vi "GreaseTestingByAleks.vi"() -> ()   [LabVIEW 2021]
uses:
  <vilib>/Utility/error.llb/DialogType.ctl
  <vilib>/DAQmx/read.llb/DAQmx Read (Analog 2D DBL NChan NSamp).vi
  <vilib>/Analysis/baseanly.llb/A x Vector.vi
  <vilib>/DAQmx/create/channels.llb/DAQmx Create Channel (AI-Voltage-Basic).vi
  <vilib>/DAQmx/configure/timing.llb/DAQmx Timing (Sample Clock).vi
  <vilib>/DAQmx/miscellaneous.llb/DAQmx Fill In Error Info.vi
  <vilib>/Utility/file.llb/Write To Spreadsheet File (DBL).vi
  <vilib>/Utility/file.llb/Read Delimited Spreadsheet (string).vi
  Zaber A Series/Zaber A Series.lvlib
  <vilib>/Analysis/NI_AALBase.lvlib
panel:
  out "Force Units 2":string
  out "Torque Units 2":string
  in  "Transform":T1
  out "Calibration Matrix":dbl[][](array[numeric])
  out "Voltages":dbl[][](array[numeric])
  out "F/T":dbl[][](array[numeric]) format="%0.2f"
  out "Bias Voltages":dbl[][](array[numeric])
  out "Bias Vector":dbl[](array[numeric])
  in  "Setting":string(combo)
  out "Command Responses":string[](array[string])
  in  "Data":string
  in  "Command List":string(combo)
  in  "Value to Send":string
  out "Current Value":string
  in  "Send Command":bool
  in  "Get Setting":bool
  in  "Change Setting":bool
  in  "Torque Units":string
  in  "Force Units":string
  in  "Calibration File":path
  in  "First Channel":i16
  in  "DAQ Card":tag
  in  "Samples to Read":i32=1000
  in  "stop":bool
  out "Measurement":dbl[][](graph) caption="F/T Data"
  in  "Bias":bool
  in  "Unbias":bool
  in  "Collect Data":bool=TRUE
  in  "Data File":path
  in  "Maximum Value":dbl=10.0 format="%0.2f"
  in  "Minimum Value":dbl=-10.0 format="%0.2f"
  in  "Sample Rate":dbl=10000.0 caption="Sample Rate (Hz)" format="%0.2f"
  in  "Units (0: microsteps)":u16(ring) items=["microsteps", "microns", "millimeters", "inches"]
  in  "Device Number & Axis":string(combo)
  in  "Microstep Size (0)":dbl
  out "Device Number\n& Axis":string[](array[string])
  out "Model Name":string[](array[string])
  out "Microstep\nSize":dbl[](array[numeric])
  out "Motion Type":string[](array[string])
  in  "Move Distance (0)":dbl format="%#_12f"
  in  "Movement Type (0: relative)":u16(ring) items=["relative", "absolute"]
  in  "VISA resource name":refnum<visa-resource-name>
  in  "Start Tracking":bool
  out "Position":dbl format="%#_15f"
  in  "Identify Devices":bool
  in  "Close Port":bool
  in  "Execute Movement":bool
  in  "Home":bool
  in  "Open Port":bool
  # "Greases Control Panel"
  # "Things Aleks is Not Sure About"
  # "Force Sensor Things That Aleks Doesn't Understand"
  # "Send Command"
  # "Read and Modify Settings"
  # "Setup"
  # "Running"
  # "Motor Control Port Settings"
  # "Force Sensor DAQ Settings"
  # "Force Sensor File Settings"
  # "Force Sensor Output and Controls"
  # "Identify Connected Devices"
  # "Send Movement"
  # "Don't Collect Data"
  # "Motor Shared Settings"
  # "Force Sensor Measurement Settings"
  # "Home Devices"
  # "Position Tracking"
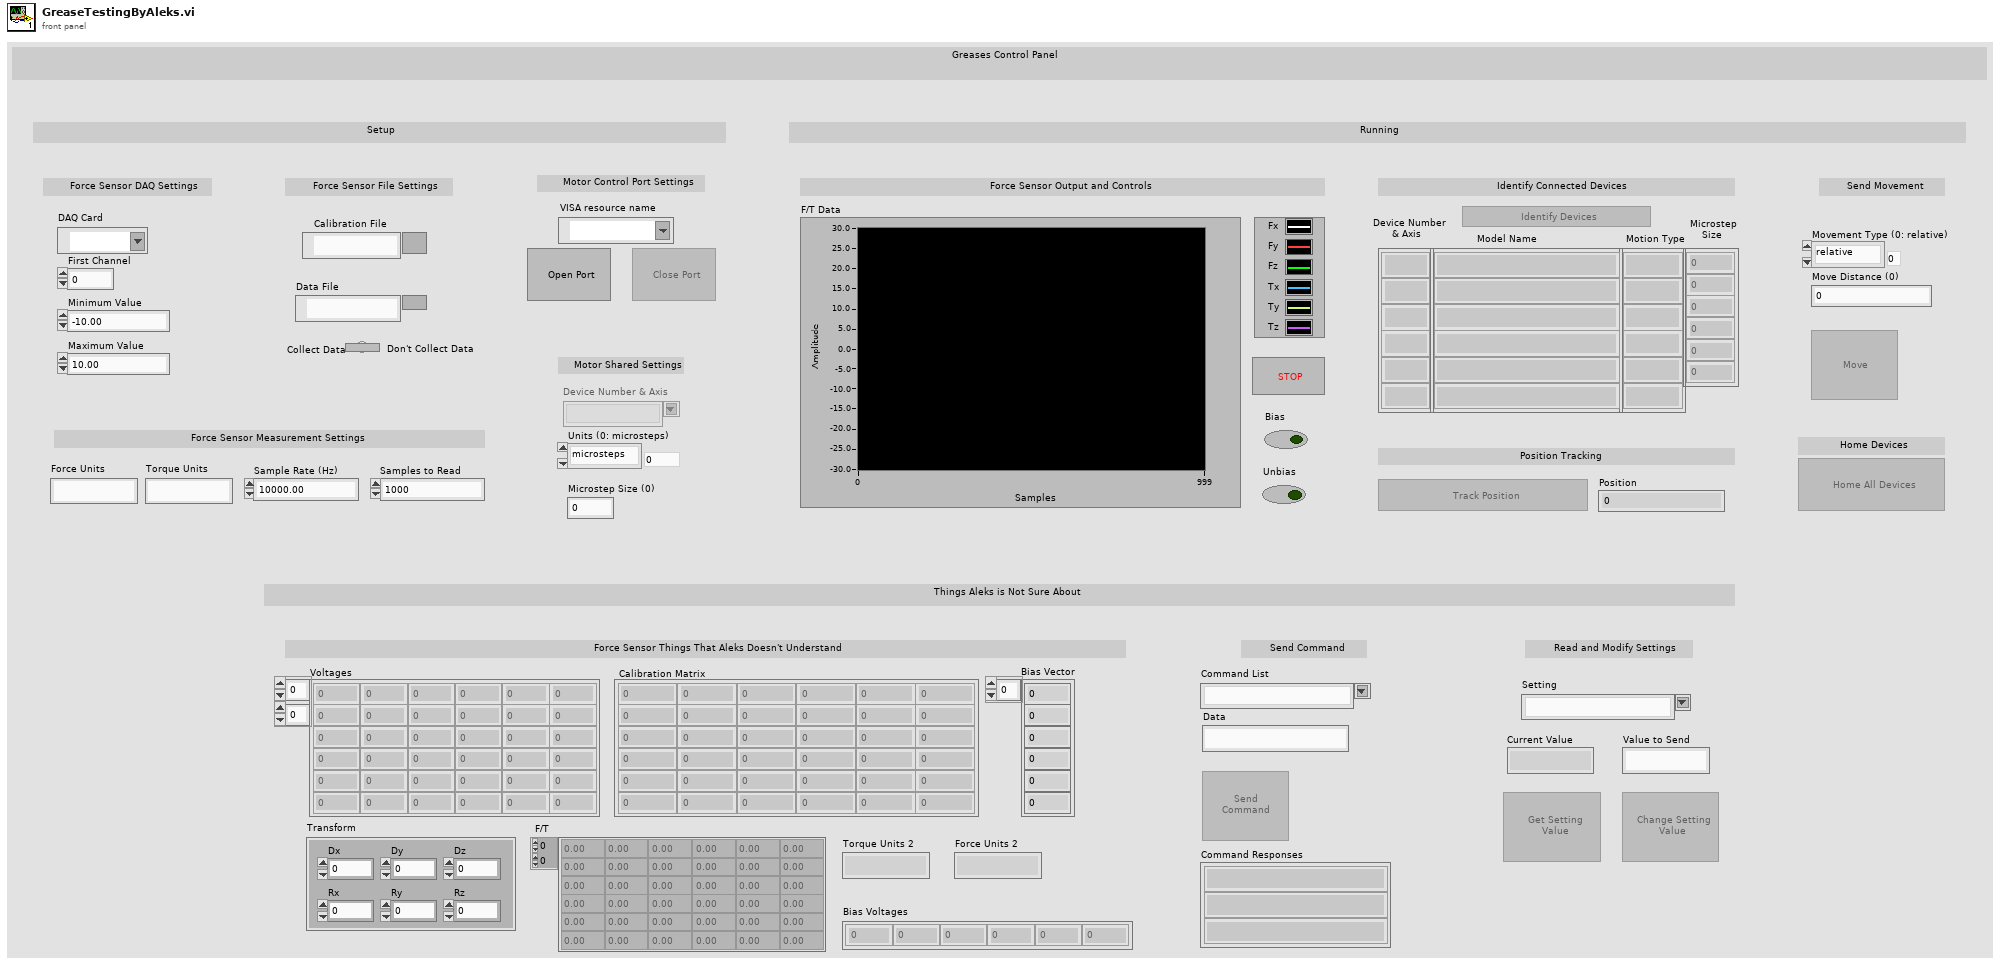
[diagram p1: front panel]
types:
  T1 = cluster{"Dx":dbl, "Dy":dbl, "Dz":dbl, "Rx":dbl, "Ry":dbl, "Rz":dbl}
  T2 = typedef "DialogType.ctl" = u16
  T3 = enum8{"Enabled", "Disabled", "Disabled and Grayed Out"}
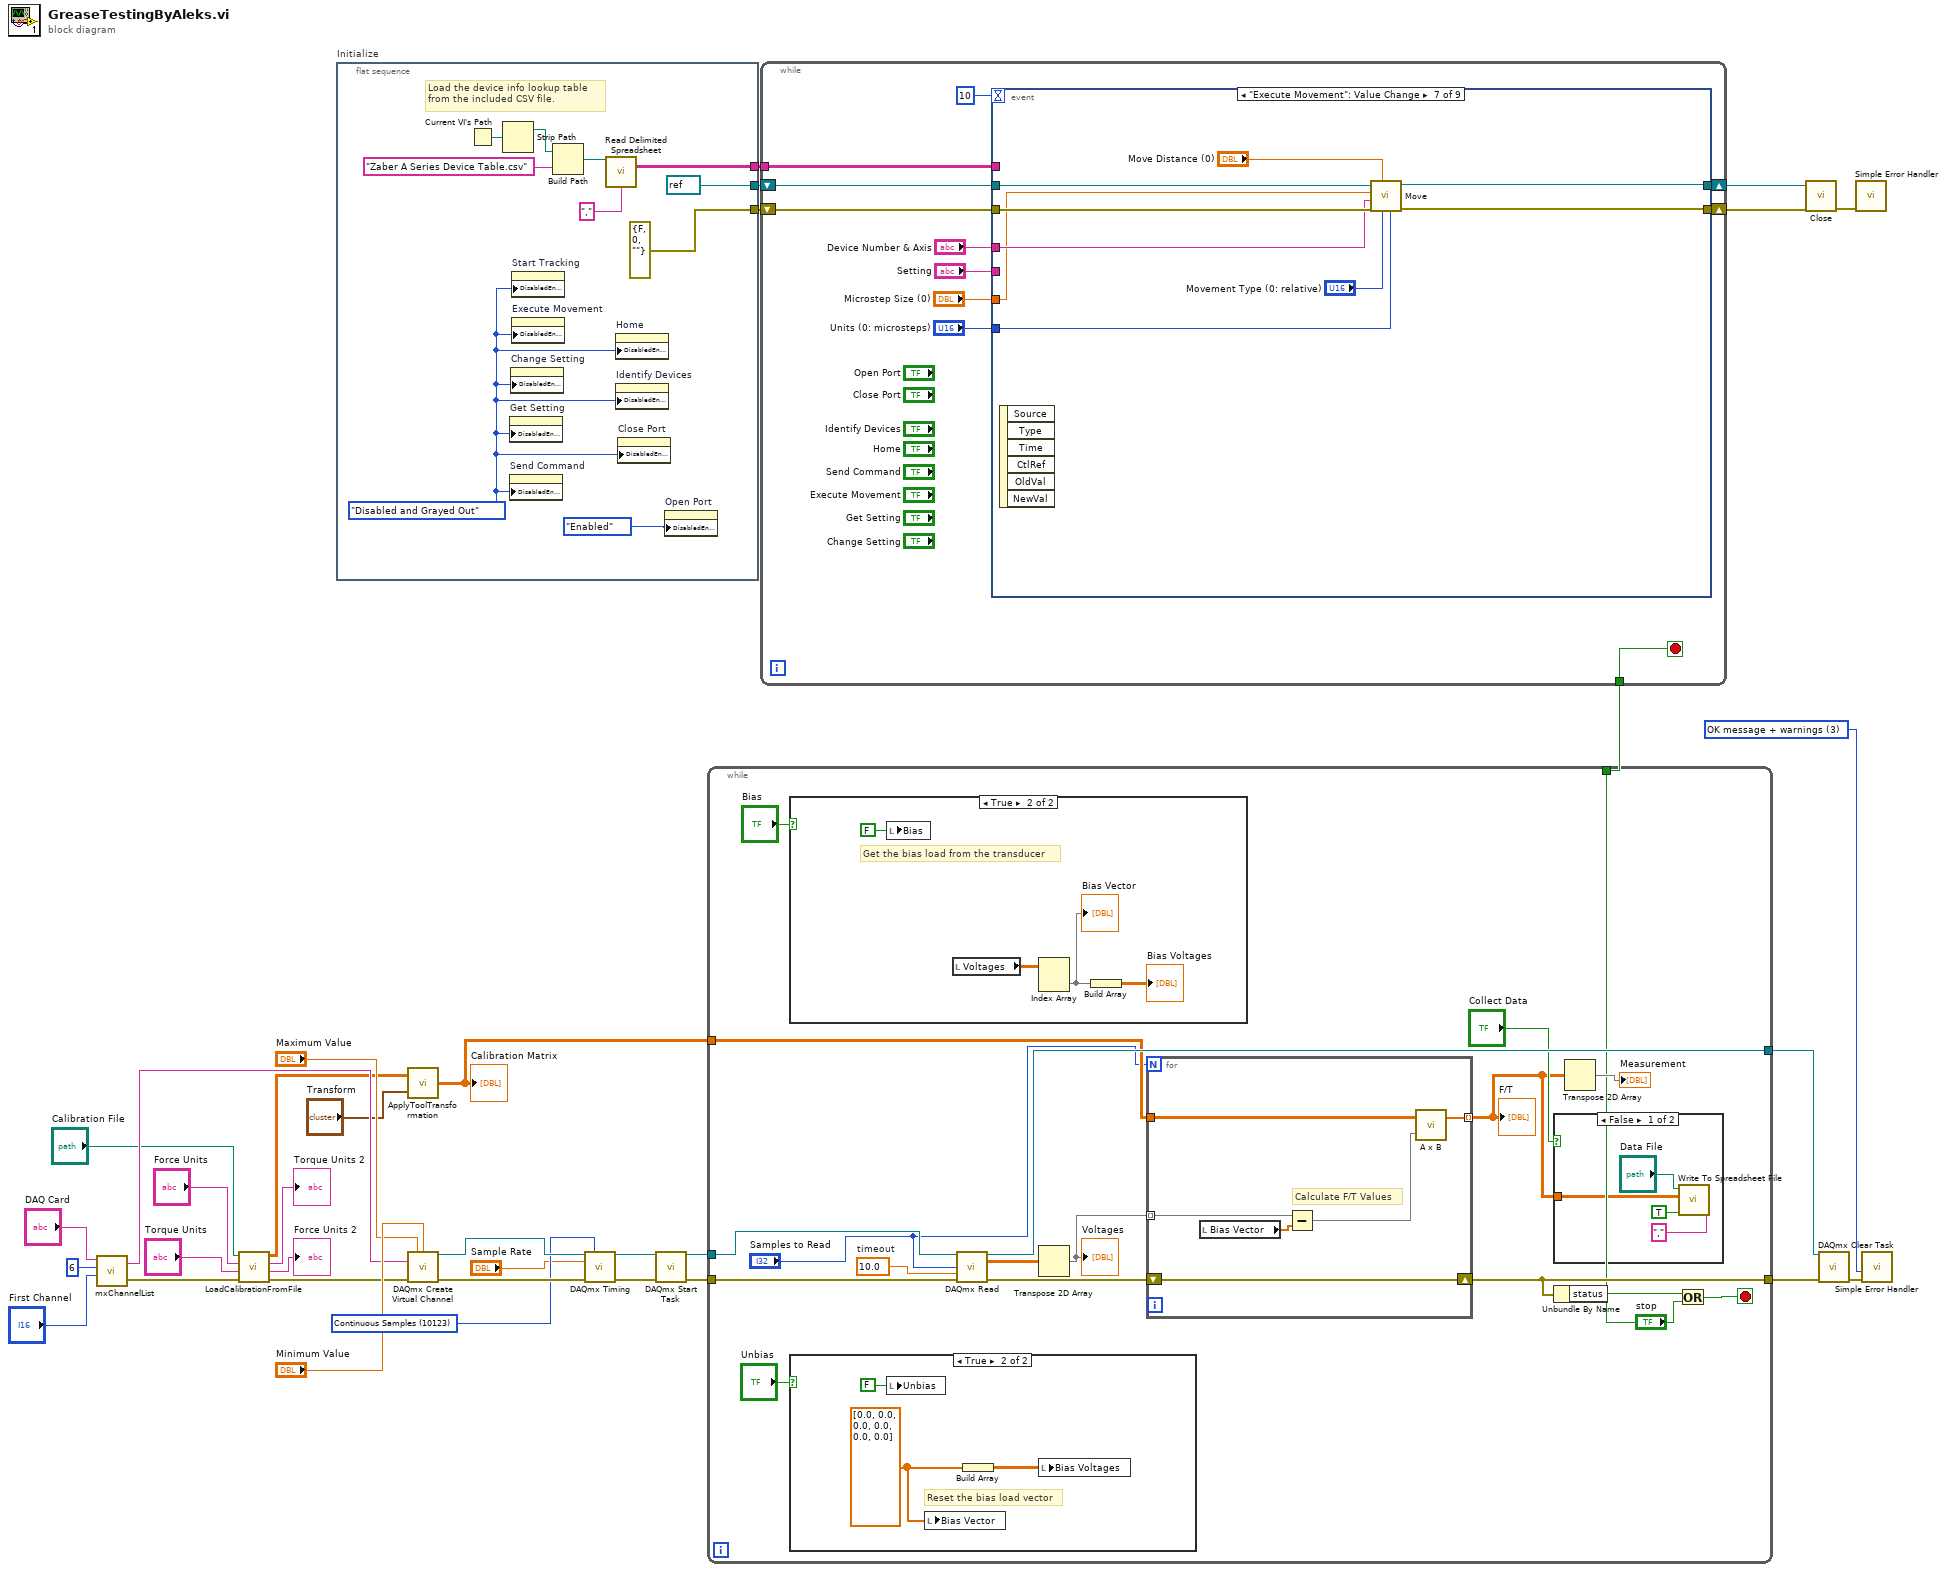
[diagram p0: block diagram]
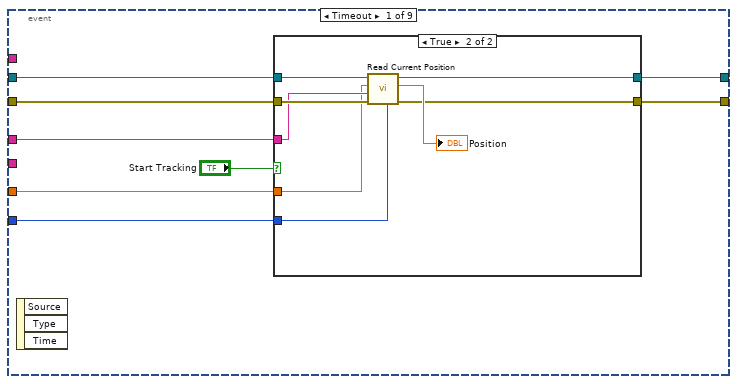
[diagram p5: hidden frame]
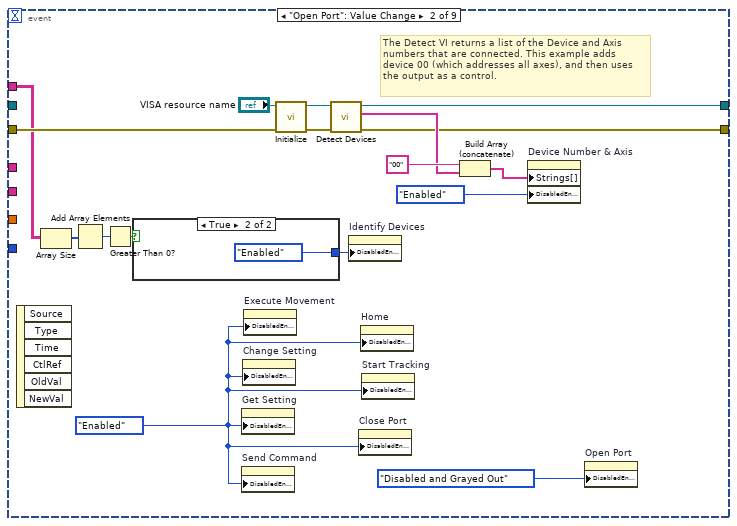
[diagram p7: hidden frame]
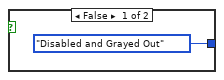
[diagram p8: hidden frame]
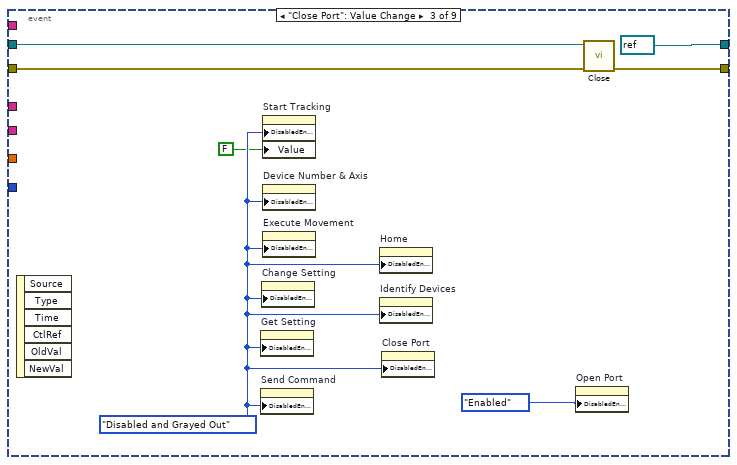
[diagram p9: hidden frame]
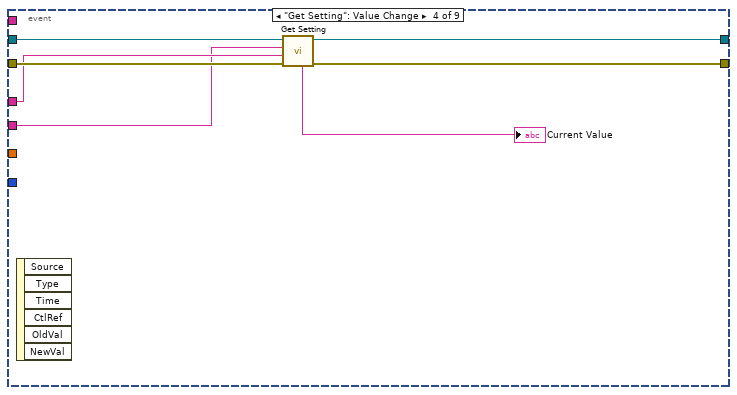
[diagram p10: hidden frame]
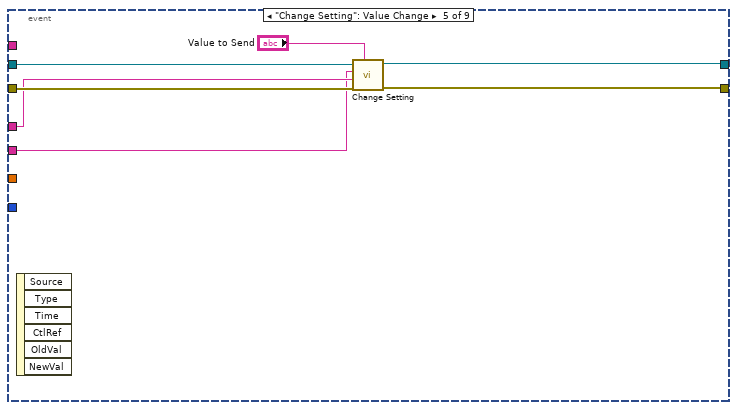
[diagram p11: hidden frame]
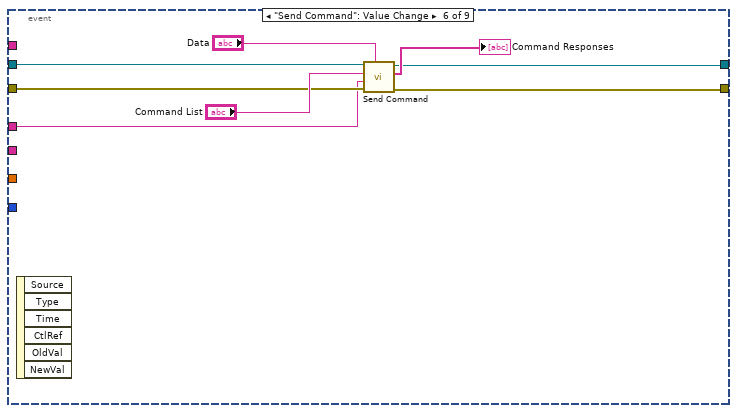
[diagram p12: hidden frame]
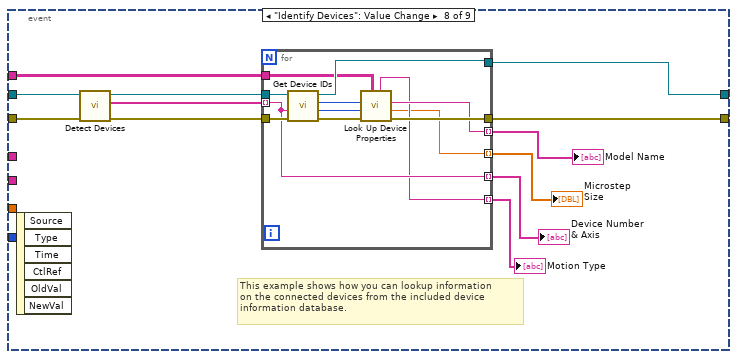
[diagram p13: hidden frame]
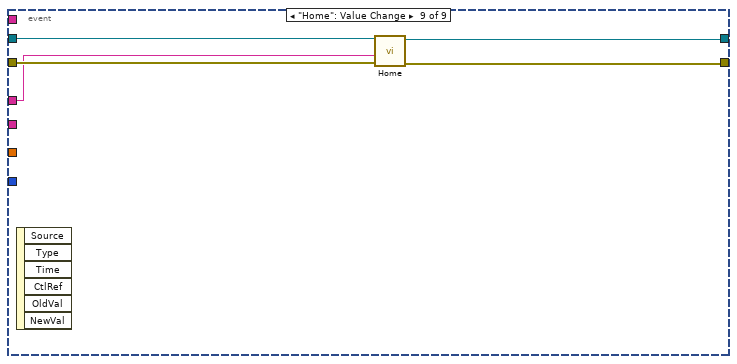
[diagram p14: hidden frame]
diagram:
  w19 = T2 3 items=["no dialog", "OK message", "continue or stop message", "OK message + warnings", "continue/stop + warnings"] ("type of dialog (OK msg:1)")
  w22 = 10123 items=["Finite Samples"=10178, "Continuous Samples"=10123] ("sample mode")
  n1 = call "mxChannelList.vi"("First Channel"="First Channel", "Number of Channels"=6, "DAQmx Device Name"="DAQ Card") -> ("error out"=w3:errorcluster, "Channel List"=w15:string)  [unwired: 1 in]
  n2 = call "LoadCalibrationFromFile.vi"("Error In"=w3, "User Torque Units"="Torque Units", "User Force Units"="Force Units", "Cal File Path"="Calibration File") -> ("Error Out"=w2:errorcluster, "Calibration Force Units"=→"Force Units 2":string, "Calibration Torque Units"=→"Torque Units 2":string, "Calibration Matrix"=w9:dbl[][])
  n3 = flat-sequence "Initialize" {
    tunnel: [errorcluster {"status"=FALSE, "code"=0, "source"=""} ("error out")] -> w35
    tunnel: [w39] -> w31
    tunnel: [refnum<visa-resource-name> refnum ("VISA resource name")] -> w30
    frame #0 {
      w36 = T3."Disabled and Grayed Out" ("Disabled")
      # "Load the device info lookup table\nfrom the included CSV file."
      n4 = Current VI's Path() -> (path=w43:path)
      n5 = Strip Path(path=w43) -> (stripped path=w44:path)  [unwired: 1 out]
      n6 = property on="Get Setting" class="Bool"("DisabledEnum"=w36) -> ()  [unwired: 2 in, 2 out]
      n7 = property on="Send Command" class="Bool"("DisabledEnum"=w36) -> ()  [unwired: 2 in, 2 out]
      n8 = property on="Change Setting" class="Bool"("DisabledEnum"=w36) -> ()  [unwired: 2 in, 2 out]
      n9 = property on="Start Tracking" class="Bool (strict)"("DisabledEnum"=w36) -> ()  [unwired: 2 in, 2 out]
      n10 = property on="Execute Movement" class="Bool"("DisabledEnum"=w36) -> ()  [unwired: 2 in, 2 out]
      n11 = Build Path(base path=w44, name or relative path="Zaber A Series Device Table.csv") -> (appended path=w41:path)
      n12 = call-poly <vilib>:"Read Delimited Spreadsheet.vi"("file path (dialog if empty)"=w41, "delimiter (\\t)"="," ("delimiter (\\t)")) -> ("all rows"=w39:string[][])  [unwired: 8 in, 5 out]
      n13 = property on="Home" class="Bool"("DisabledEnum"=w36) -> ()  [unwired: 2 in, 2 out]
      n14 = property on="Identify Devices" class="Bool"("DisabledEnum"=w36) -> ()  [unwired: 2 in, 2 out]
      n15 = property on="Close Port" class="Bool"("DisabledEnum"=w36) -> ()  [unwired: 2 in, 2 out]
      n16 = property on="Open Port" class="Bool"("DisabledEnum"=T3."Enabled" ("Disabled")) -> ()  [unwired: 2 in, 2 out]
    }
  }
  n17 = call "ApplyToolTransformation.vi"("Transform"="Transform", "Calibration Matrix"=w9) -> ("Transformed Calibration Matrix"=w8:dbl[][])
  "Calibration Matrix" <- w8
  n18 = call-poly <vilib>:"DAQmx Create Virtual Channel.vi"("maximum value"="Maximum Value", "minimum value"="Minimum Value", "physical channels"=w15, "error in"=w2) -> ("task out"=w25:refnum<k21>, "error out"=w27:errorcluster)  [unwired: 10 in]
  n19 = call-poly <vilib>:"DAQmx Timing.vi"("task/channels in"=w25, "sample mode"=w22, "rate"="Sample Rate", "error in"=w27) -> ("task out"=w21:refnum<k21>, "error out"=w14:errorcluster)  [unwired: 10 in]
  n20 = call <vilib>:"DAQmx Start Task.vi"("task/channels in"=w21, "error in"=w14) -> ("task out"=w24:refnum<k21>, "error out"=w13:errorcluster)  [unwired: 12 in]
  n21 = while {
    tunnel: w24 -> [w63]
    tunnel: [w62] -> w23
    tunnel: w13 -> [w60]
    tunnel: [w56] -> w12
    tunnel: w8 -> [w53]
    tunnel: ["stop"] -> w1
    stop <- w58 stop-if-true
    w61 = 10.0  # timeout
    n22 = case shown="True" "Bias" {
      frame False {
      }
      frame True {
        # "Get the bias load from the transducer"
        n23 = local write "Bias"(FALSE) -> ()
        n24 = local read "Voltages"() -> (w74:dbl[][])
        n25 = Index Array(array=w74) -> (element=w73:dbl[])  [unwired: 2 in]
        "Bias Vector" <- w73
        n26 = Build Array(w73) -> (→"Bias Voltages":dbl[][])
      }
    }
    n27 = case shown="True" "Unbias" {
      frame False {
      }
      frame True {
        w69 = dbl[] [0.0, 0.0, 0.0, 0.0, 0.0, 0.0]
        # "Reset the bias load vector"
        n28 = local write "Unbias"(FALSE) -> ()
        n29 = local write "Bias Vector"(w69) -> ()
        n30 = Build Array(w69) -> (w68:dbl[][])
        n31 = local write "Bias Voltages"(w68) -> ()
      }
    }
    n32 = call-poly <vilib>:"DAQmx Read.vi"("task/channels in"=w63, "number of samples per channel"="Samples to Read", "timeout"=w61, "error in"=w60) -> ("task out"=w62:refnum<k21>, "data"=w55:dbl[][], "error out"=w57:errorcluster)  [unwired: 9 in]
    n33 = Transpose 2D Array(2D array=w55) -> (transposed array=w51:dbl[][])
    "Voltages" <- w51
    n34 = for {
      N: "Samples to Read" -> [_]
      tunnel: [w77] -> w47 mode=indexing
      shift-right: [w76] -> w56
      shift-left: w57 -> [w76]
      tunnel: w51 -> [w80] mode=indexing
      tunnel: w53 -> [w75]
      # "Calculate F/T Values"
      n35 = local read "Bias Vector"() -> (w79:dbl[])
      n36 = Subtract(x=w80, y=w79) -> (x-y=w78:dbl[])
      n37 = call-poly <vilib>:"A x B.vi"("Vector"=w78, "A"=w75) -> ("A x Vector"=w77:dbl[])  [unwired: 1 out]
    }
    "F/T" <- w47
    n38 = case shown="False" "Collect Data" {
      tunnel: w47 -> [w67 _]
      frame False {
        n39 = call-poly <vilib>:"Write To Spreadsheet File.vi"("delimiter (\\t)"=",", "append to file? (new file:F)"=TRUE, "2D data"=w67, "file path (dialog if empty)"="Data File") -> ()  [unwired: 4 in, 1 out]
      }
      frame True {
      }
    }
    n40 = Unbundle By Name(w56) -> ("status"=w59:bool)
    n41 = Transpose 2D Array(2D array=w47) -> (transposed array=→"Measurement":dbl[][])
    n42 = Or(x=w59, y="stop") -> (x .or. y?=w58:bool)
  }
  n43 = while {
    shift-right: [w87] -> w34
    shift-left: w30 -> [w89]
    shift-right: [w86] -> w33
    shift-left: w35 -> [w88]
    tunnel: w31 -> [w90]
    tunnel: w1 -> [w81]
    stop <- w81 stop-if-true
    n44 = event shown="[6] \"Execute Movement\": Value Change" {
      selector: _ -> [_ _ _ _ _ _ _ _ _]
      dyn-events: _ -> [_ _ _ _ _ _ _ _ _]
      timeout: u32 10 ("milliseconds to wait") -> [_ _ _ _ _ _ _ _ _]
      tunnel: w90 -> [_ w114 _ _ _ _ _ w167 _]
      tunnel: w89 -> [w98 _ w135 w142 w148 w154 w164 w171 w195]
      tunnel: w88 -> [w97 w119 w134 w141 w146 w153 w163 w170 w193]
      tunnel: [w95 w118 w132 w139 w145 w152 w162 w168 w192] -> w86
      tunnel: [w96 w117 refnum<visa-resource-name> refnum ("VISA resource name") w140 w147 w151 w161 w169 w194] -> w87
      tunnel: "Device Number & Axis" -> [w94 _ _ w138 w144 w150 w160 _ w191]
      tunnel: "Setting" -> [_ _ _ w137 w143 _ _ _ _]
      tunnel: "Microstep Size (0)" -> [w93 _ _ _ _ _ w159 _ _]
      tunnel: "Units (0: microsteps)" -> [w92 _ _ _ _ _ w158 _ _]
      event Timeout {
        n45 = event-data() -> ()  [unwired: 1 in, 3 out]
        n46 = case shown="True" "Start Tracking" {
          tunnel: w98 -> [w101 w108]
          tunnel: w97 -> [w100 w106]
          tunnel: [w101 w107] -> w96
          tunnel: [w100 w105] -> w95
          tunnel: w94 -> [_ w104]
          tunnel: w93 -> [_ w103]
          tunnel: w92 -> [_ w102]
          frame False {
          }
          frame True {
            n47 = call "Read Current Position.vi"("Units (0: microsteps)"=w102, "error in (no error)"=w106, "Device and Axis"=w104, "Microstep Size (0)"=w103, "VISA resource name"=w108) -> ("error out"=w105:errorcluster, "Position"=→"Position":dbl, "VISA resource name out"=w107:refnum<visa-resource-name>)  [unwired: 4 in]
          }
        }
      }
      event "Open Port": Value Change {
        w115 = T3."Enabled" ("Disabled")
        # "The Detect VI returns a list of the Device and Axis\nnumbers that are connected. This example adds\ndevice 00 (which addresses all axes), and then uses\nthe output as a control."
        n48 = event-data() -> ()  [unwired: 1 in, 6 out]
        n49 = Array Size(array=w114) -> (size(s)=w113:i32[])
        n50 = Add Array Elements(numeric array=w113) -> (sum=w112:i32)
        n51 = Greater Than 0?(x=w112) -> (x > 0?=w111:bool)
        n52 = case shown="True" w111 {
          tunnel: [T3."Disabled and Grayed Out" ("Disabled") T3."Enabled" ("Disabled")] -> w110
          frame False {
          }
          frame True {
          }
        }
        n53 = property on="Get Setting" class="Bool"("DisabledEnum"=w115) -> ()  [unwired: 2 in, 2 out]
        n54 = property on="Send Command" class="Bool"("DisabledEnum"=w115) -> ()  [unwired: 2 in, 2 out]
        n55 = property on="Change Setting" class="Bool"("DisabledEnum"=w115) -> ()  [unwired: 2 in, 2 out]
        n56 = property on="Execute Movement" class="Bool"("DisabledEnum"=w115) -> ()  [unwired: 2 in, 2 out]
        n57 = call "Initialize.vi"("error in (no error)"=w119, "VISA resource name"="VISA resource name") -> ("error out"=w122:errorcluster, "VISA resource name out"=w121:refnum<visa-resource-name>)  [unwired: 8 in]
        n58 = call "Detect Devices.vi"("error in (no error)"=w122, "VISA resource name"=w121) -> ("error out"=w118:errorcluster, "Connected Devices and Axes"=w124:string[], "VISA resource name out"=w117:refnum<visa-resource-name>)  [unwired: 6 in, 1 out]
        n59 = property on="Identify Devices" class="Bool"("DisabledEnum"=w110) -> ()  [unwired: 2 in, 2 out]
        n60 = property on="Close Port" class="Bool"("DisabledEnum"=w115) -> ()  [unwired: 2 in, 2 out]
        n61 = property on="Home" class="Bool"("DisabledEnum"=w115) -> ()  [unwired: 2 in, 2 out]
        n62 = property on="Start Tracking" class="Bool (strict)"("DisabledEnum"=w115) -> ()  [unwired: 2 in, 2 out]
        n63 = Build Array (concatenate)("00", w124) -> (w125:string[])
        n64 = property on="Device Number & Axis" class="CmbBox"("Strings[]"=w125, "DisabledEnum"=T3."Enabled" ("Disabled")) -> ()  [unwired: 2 in, 2 out]
        n65 = property on="Open Port" class="Bool"("DisabledEnum"=T3."Disabled and Grayed Out" ("Disabled")) -> ()  [unwired: 2 in, 2 out]
      }
      event "Close Port": Value Change {
        w130 = T3."Disabled and Grayed Out" ("Disabled")
        n66 = event-data() -> ()  [unwired: 1 in, 6 out]
        n67 = property on="Get Setting" class="Bool"("DisabledEnum"=w130) -> ()  [unwired: 2 in, 2 out]
        n68 = property on="Send Command" class="Bool"("DisabledEnum"=w130) -> ()  [unwired: 2 in, 2 out]
        n69 = property on="Change Setting" class="Bool"("DisabledEnum"=w130) -> ()  [unwired: 2 in, 2 out]
        n70 = property on="Start Tracking" class="Bool (strict)"("DisabledEnum"=w130, "Value"=FALSE ("Start Tracking")) -> ()  [unwired: 2 in, 2 out]
        n71 = property on="Device Number & Axis" class="CmbBox"("DisabledEnum"=w130) -> ()  [unwired: 2 in, 2 out]
        n72 = property on="Execute Movement" class="Bool"("DisabledEnum"=w130) -> ()  [unwired: 2 in, 2 out]
        n73 = property on="Home" class="Bool"("DisabledEnum"=w130) -> ()  [unwired: 2 in, 2 out]
        n74 = property on="Identify Devices" class="Bool"("DisabledEnum"=w130) -> ()  [unwired: 2 in, 2 out]
        n75 = property on="Close Port" class="Bool"("DisabledEnum"=w130) -> ()  [unwired: 2 in, 2 out]
        n76 = property on="Open Port" class="Bool"("DisabledEnum"=T3."Enabled" ("Disabled")) -> ()  [unwired: 2 in, 2 out]
        n77 = call "Close.vi"("error in (no error)"=w134, "VISA resource name"=w135) -> ("error out"=w132:errorcluster)  [unwired: 9 in]
      }
      event "Get Setting": Value Change {
        n78 = event-data() -> ()  [unwired: 1 in, 6 out]
        n79 = call "Get Setting.vi"("error in (no error)"=w141, "Device and Axis"=w138, "Setting"=w137, "VISA resource name"=w142) -> ("error out"=w139:errorcluster, "VISA resource name out"=w140:refnum<visa-resource-name>, "First Response Data"=→"Current Value":string)  [unwired: 2 in, 3 out]
      }
      event "Change Setting": Value Change {
        n80 = event-data() -> ()  [unwired: 1 in, 6 out]
        n81 = call "Change Setting.vi"("Data"="Value to Send", "error in (no error)"=w146, "Device and Axis"=w144, "Setting"=w143, "VISA resource name"=w148) -> ("error out"=w145:errorcluster, "VISA resource name out"=w147:refnum<visa-resource-name>)  [unwired: 5 in]
      }
      event "Send Command": Value Change {
        n82 = event-data() -> ()  [unwired: 1 in, 6 out]
        n83 = call "Send Command.vi"("Data"="Data", "error in (no error)"=w153, "Device and Axis"=w150, "Command"="Command List", "VISA resource name"=w154) -> ("error out"=w152:errorcluster, "Response String Array"=→"Command Responses":string[], "VISA resource name out"=w151:refnum<visa-resource-name>)  [unwired: 1 in, 3 out]
      }
      event "Execute Movement": Value Change {
        n84 = event-data() -> ()  [unwired: 1 in, 6 out]
        n85 = call "Move.vi"("Units (0: microsteps)"=w158, "Movement Type (0: relative)"="Movement Type (0: relative)", "Move Distance (0)"="Move Distance (0)", "error in (no error)"=w163, "Device and Axis"=w160, "Microstep Size (0)"=w159, "VISA resource name"=w164) -> ("error out"=w162:errorcluster, "VISA resource name out"=w161:refnum<visa-resource-name>)  [unwired: 3 in]
      }
      event "Identify Devices": Value Change {
        # "This example shows how you can lookup information\non the connected devices from the included device \ninformation database."
        n86 = event-data() -> ()  [unwired: 1 in, 6 out]
        n87 = call "Detect Devices.vi"("error in (no error)"=w170, "VISA resource name"=w171) -> ("error out"=w173:errorcluster, "Connected Devices and Axes"=w174:string[], "VISA resource name out"=w172:refnum<visa-resource-name>)  [unwired: 6 in, 1 out]
        n88 = for {
          tunnel: w172 -> [w190]
          tunnel: w173 -> [w189]
          tunnel: [w185] -> w168
          tunnel: w174 -> [w184] mode=indexing
          tunnel: [w184] -> w175 mode=indexing
          tunnel: [w183] -> w176 mode=indexing
          tunnel: [w179] -> w177 mode=indexing
          tunnel: [w182] -> w178 mode=indexing
          tunnel: [w181] -> w169
          tunnel: w167 -> [w180]
          n89 = call "Get Device IDs.vi"("error in (no error)"=w189, "Device and Axis"=w184, "VISA resource name"=w190) -> ("error out"=w186:errorcluster, "Peripheral ID"=w187:i32, "Device ID"=w188:i32, "VISA resource name out"=w181:refnum<visa-resource-name>)  [unwired: 5 in]
          n90 = call "Look Up Device Properties.vi"("Lookup Table"=w180, "error in (no error)"=w186, "Peripheral ID (0)"=w187, "Device ID"=w188) -> ("error out"=w185:errorcluster, "Microstep Size"=w179:dbl, "Device Name"=w183:string, "Motion Type"=w182:string)  [unwired: 4 in]
        }
        "Device Number\n& Axis" <- w175
        "Model Name" <- w176
        "Microstep\nSize" <- w177
        "Motion Type" <- w178
      }
      event "Home": Value Change {
        n91 = event-data() -> ()  [unwired: 1 in, 6 out]
        n92 = call "Home.vi"("error in (no error)"=w193, "Device and Axis"=w191, "VISA resource name"=w195) -> ("error out"=w192:errorcluster, "VISA resource name out"=w194:refnum<visa-resource-name>)  [unwired: 7 in]
      }
    }
  }
  n93 = call "Close.vi"("error in (no error)"=w33, "VISA resource name"=w34) -> ("error out"=w32:errorcluster)  [unwired: 9 in]
  n94 = call <vilib>:"DAQmx Clear Task.vi"("task in"=w23, "error in"=w12) -> ("error out"=w26:errorcluster)  [unwired: 13 in]
  n95 = call <vilib>:"Simple Error Handler.vi"("error in (no error)"=w32) -> ()  [unwired: 4 in, 5 out]
  n96 = call <vilib>:"Simple Error Handler.vi"("type of dialog (OK msg:1)"=w19, "error in (no error)"=w26) -> ()  [unwired: 3 in, 5 out]
